vi "mt_dash.vi"() -> ()   [LabVIEW 2022 SP3]
panel:
  out "Load":string[][](array[string])
  out "Process":string[][](array[string])
  in  "停止":bool
  in  "布尔":bool
  in  "数值":dbl
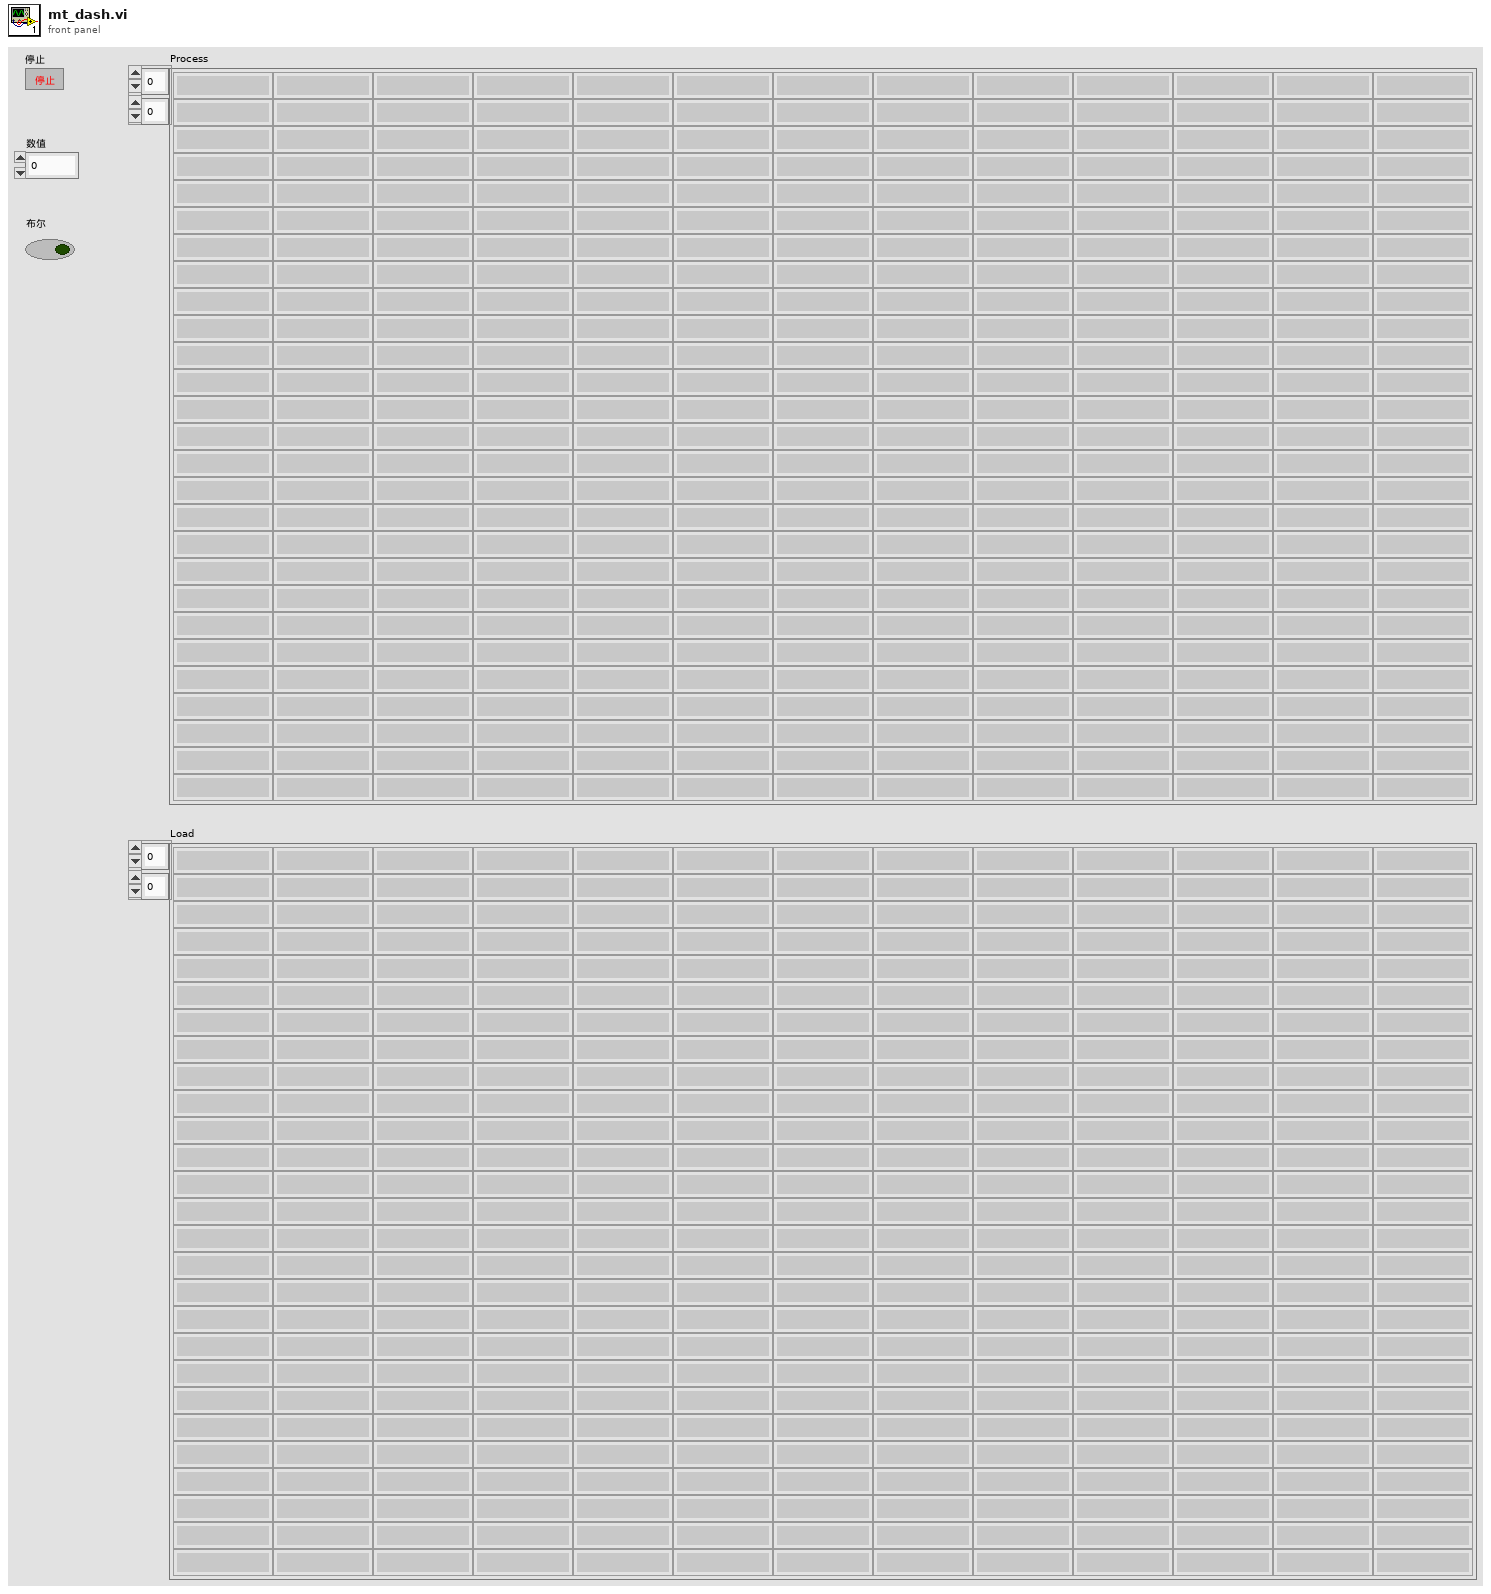
[diagram p1: front panel]
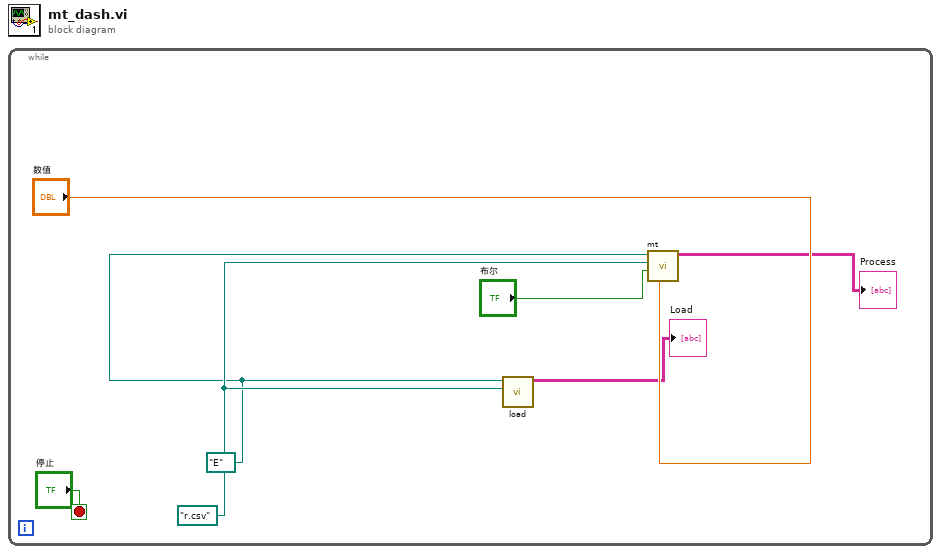
[diagram p0: block diagram]
diagram:
  n1 = while {
    stop <- "停止" stop-if-true
    w3 = path "r.csv" ("名称或相对路径")
    w2 = path "E:/" ("基路径")
    n2 = call "load.vi"("名称或相对路径"=w3, "基路径"=w2) -> ("数组"=→"Load":string[][])  [unwired: 9 in]
    n3 = call "mt.vi"("数值"="数值", "布尔"="布尔", "名称或相对路径"=w3, "基路径"=w2) -> ("数组"=→"Process":string[][])  [unwired: 7 in]
  }
